vi "Pos Controller.vi"(8 "error in (no error)":errorcluster, 10 "Notifiers":T1, 11 "All Message Queue Cluster":T2) -> (0 "error out":errorcluster)   [LabVIEW 2017]
uses:
  Lib QMH/AllMessageQueue Cluster.ctl
  Lib QMH/Message Cluster.ctl
  Lib Notifier/Notifier.ctl
  Lib QMH/MessageQueues.lvlib
  Lib Log/Logging.lvlib
  Lib Notifier/Notifier.lvlib
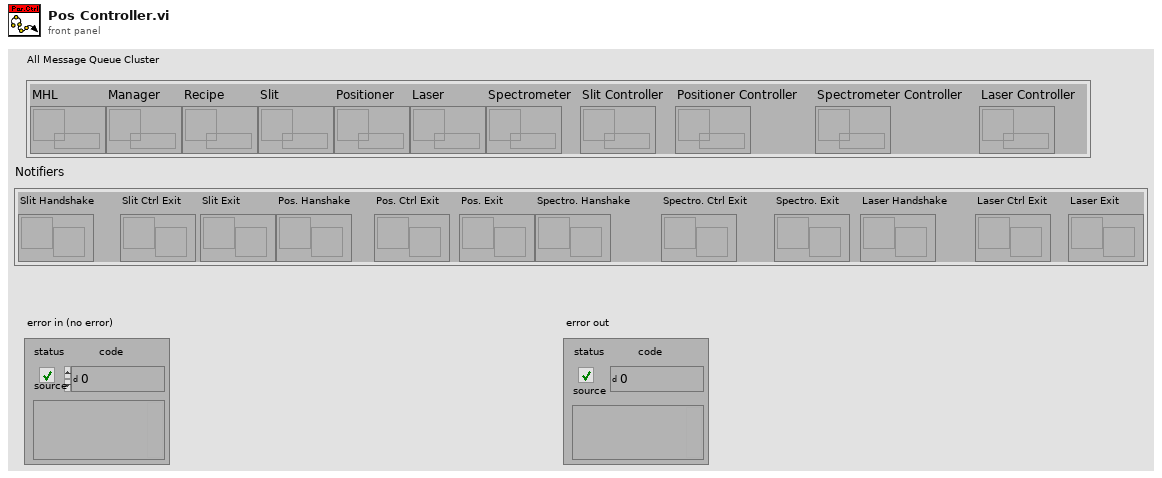
[diagram p1: front panel]
types:
  T1 = typedef "Notifier.lvlib/Notifier.ctl" = cluster{"Slit Handshake":refnum<notifier>, "Slit Ctrl Exit":refnum<notifier>, "Slit Exit":refnum<notifier>, "Pos. Hanshake":refnum<notifier>, "Pos. Ctrl Exit":refnum<notifier>, "Pos. Exit":refnum<notifier>, "Spectro. Hanshake":refnum<notifier>, "Spectro. Ctrl Exit":refnum<notifier>, "Spectro. Exit":refnum<notifier>, "Laser Handshake":refnum<notifier>, "Laser Ctrl Exit":refnum<notifier>, "Laser Exit":refnum<notifier>}
  T2 = typedef "MessageQueues.lvlib/AllMessageQueue Cluster.ctl" = cluster{"MHL":refnum<queue>, "Manager":refnum<queue>, "Recipe":refnum<queue>, "Slit":refnum<queue>, "Positioner":refnum<queue>, "Laser":refnum<queue>, "Spectrometer":refnum<queue>, "Slit Controller":refnum<queue>, "Positioner Controller":refnum<queue>, "Spectrometer Controller":refnum<queue>, "Laser Controller":refnum<queue>}
  T3 = enum16{"open", "replace", "create", "open or create", "replace or create", "replace or create with confirmation"}
  T4 = cluster{"état":bool, "code":i32, "source":string}
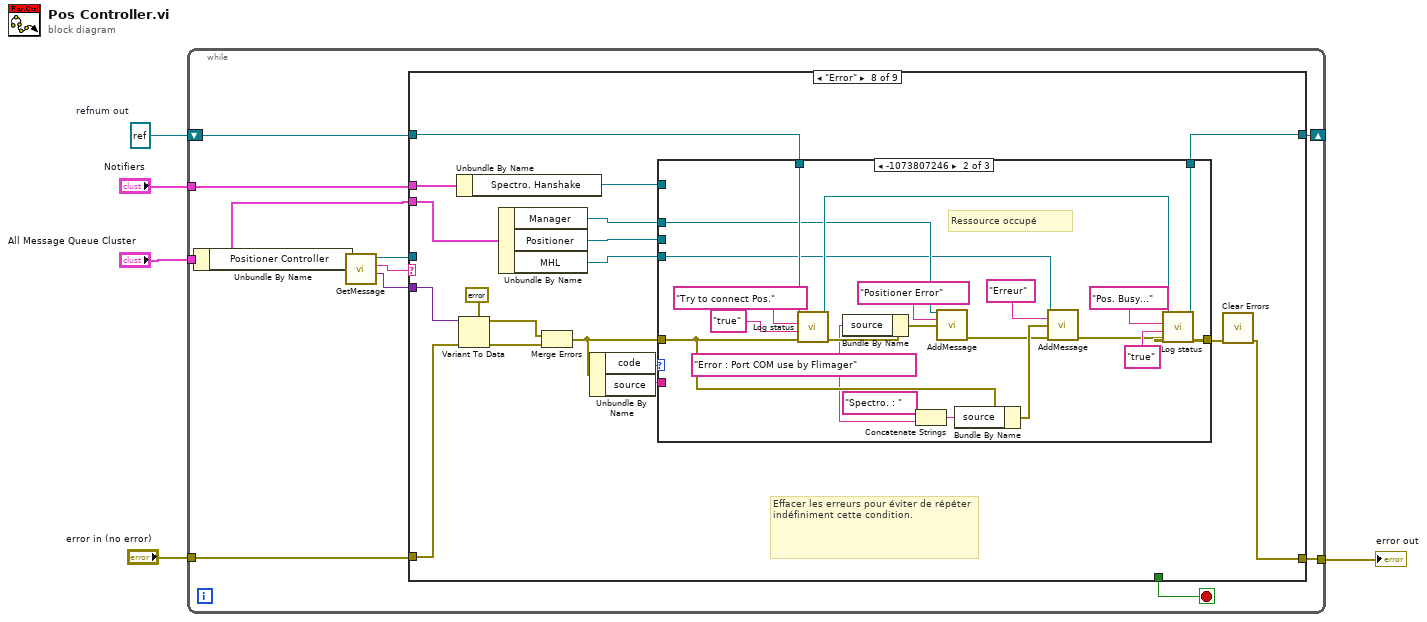
[diagram p0: block diagram]
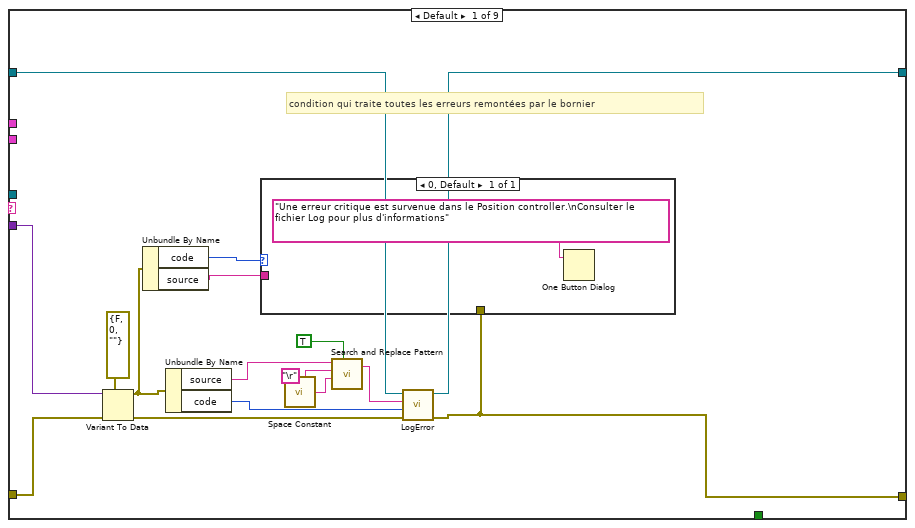
[diagram p2: hidden frame]
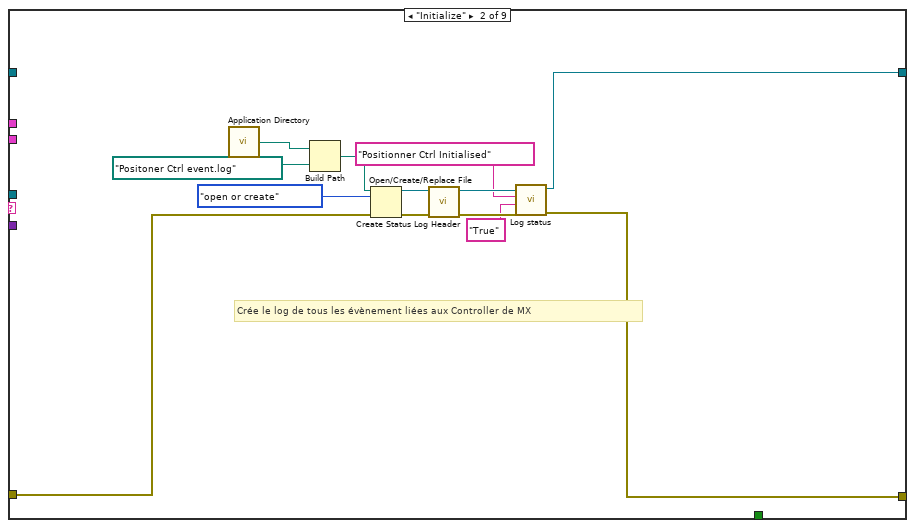
[diagram p3: hidden frame]
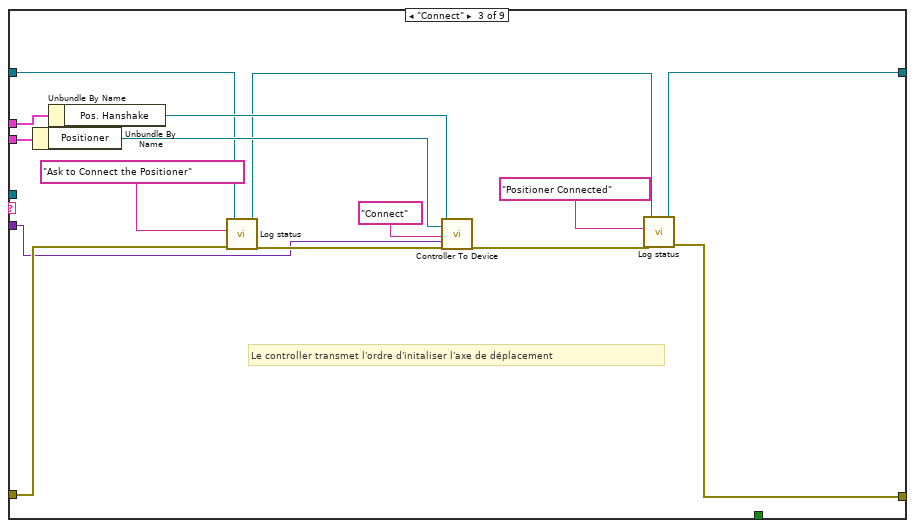
[diagram p4: hidden frame]
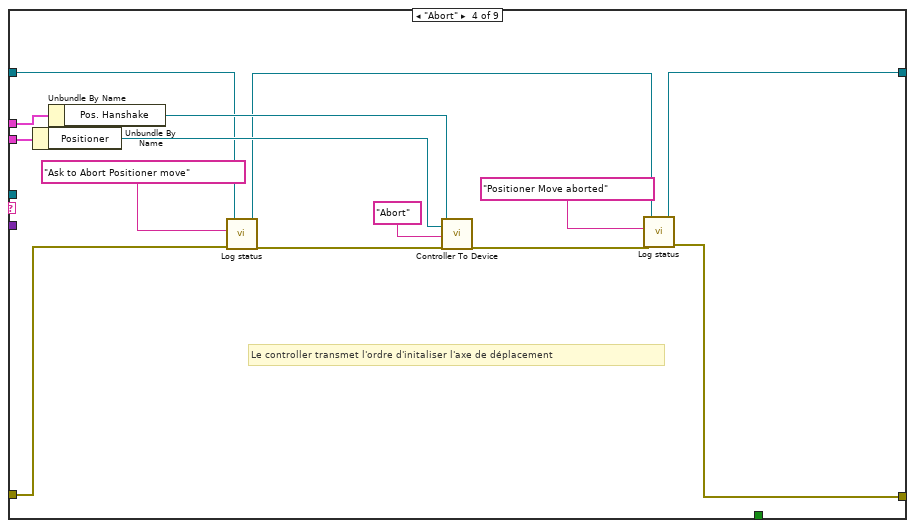
[diagram p5: hidden frame]
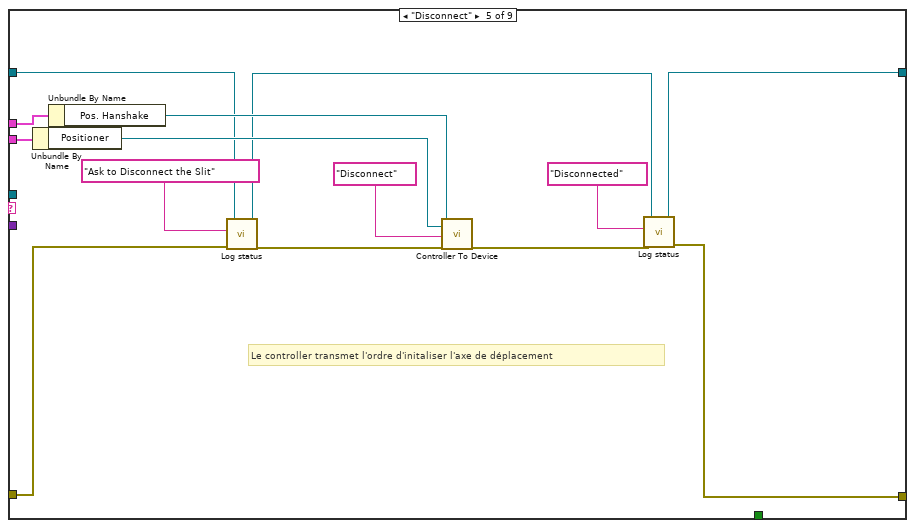
[diagram p6: hidden frame]
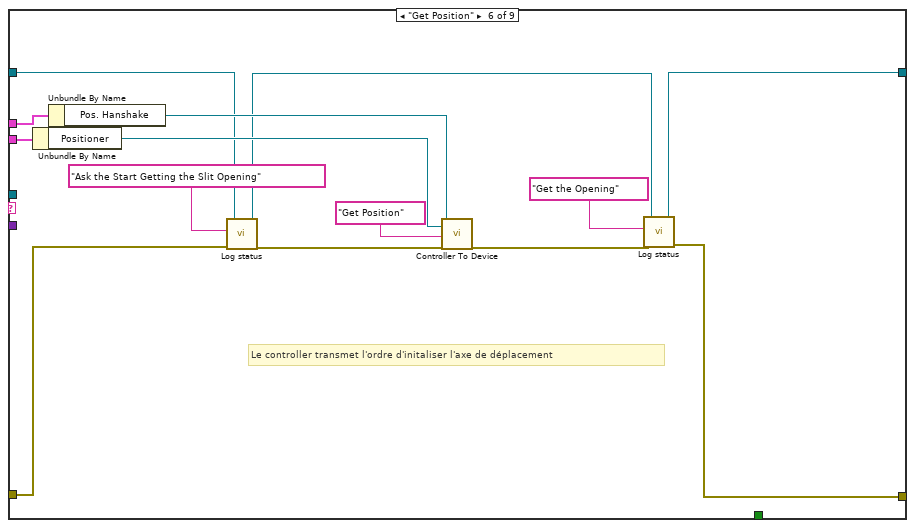
[diagram p7: hidden frame]
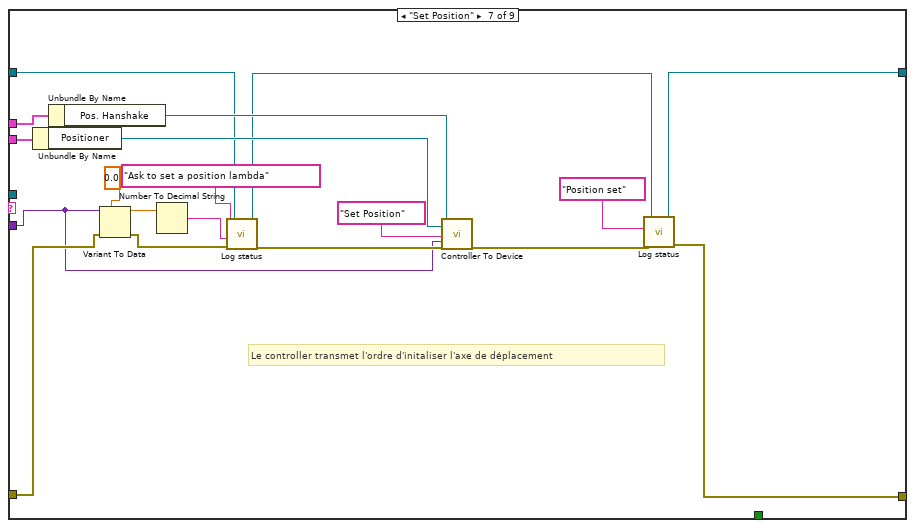
[diagram p8: hidden frame]
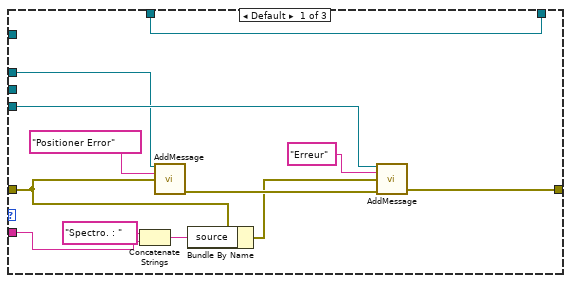
[diagram p9: hidden frame]
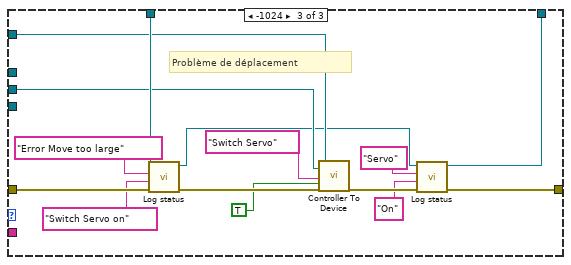
[diagram p10: hidden frame]
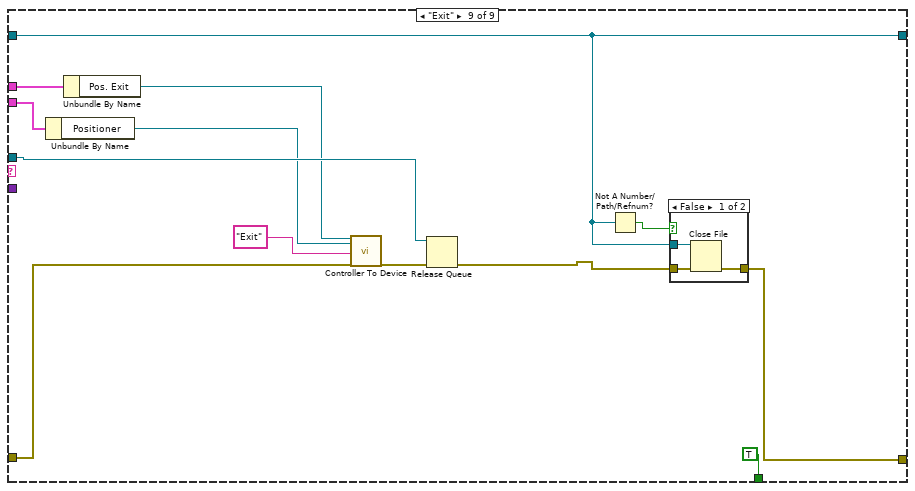
[diagram p11: hidden frame]
diagram:
  w2 = refnum<file> refnum  # refnum out
  n1 = while {
    tunnel: "All Message Queue Cluster" -> [w12]
    tunnel: "Notifiers" -> [w13]
    tunnel: "error in (no error)" -> [w8]
    tunnel: [w6] -> w1
    shift-right: [w14] -> _
    shift-left: w2 -> [w15]
    stop <- w7 stop-if-true
    n2 = Unbundle By Name(w12) -> ("Positioner Controller"=w16:refnum<queue>)
    n3 = call "GetMessage.vi"("Message queue"=w16) -> ("Data"=w9:variant, "Message"=w10:string, "Dup Message Queue"=w11:refnum<queue>)  [unwired: 7 in, 1 out]
    n4 = case shown="\"Error\"" w10 {
      tunnel: w13 -> [_ _ w61 w75 w89 w103 w122 w127 w197]
      tunnel: w12 -> [_ _ w60 w74 w88 w102 w121 w130 w196]
      tunnel: w8 -> [w21 w36 w49 w63 w77 w91 w106 w132 w192]
      tunnel: [_ _ _ _ _ _ _ _ TRUE] -> w7
      tunnel: w11 -> [_ _ _ _ _ _ _ _ w198]
      tunnel: w9 -> [w19 _ w47 _ _ _ w104 w133 _]
      tunnel: [w17 w34 w52 w66 w80 w94 w113 w125 w194] -> w14
      tunnel: w15 -> [w18 _ w56 w70 w84 w98 w117 w128 w194]
      tunnel: [w20 w35 w54 w68 w82 w96 w115 w131 w195] -> w6
      frame Default {
        # "condition qui traite toutes les erreurs remontées par le bornier"
        n5 = Variant To Data(error in=w21, type=errorcluster {"status"=FALSE, "code"=0, "source"=""} ("error in (no error)"), Variant=w19) -> (data=w32:errorcluster, error out=w23:errorcluster)
        n6 = Unbundle By Name(w32) -> ("code"=w30:i32, "source"=w31:string)
        n7 = Unbundle By Name(w32) -> ("source"=w25:string, "code"=w24:i32)
        n8 = call <vilib>:"Space Constant.vi"() -> ("String"=w27:string)
        n9 = call <vilib>:"Search and Replace Pattern.vi"("string"=w25, "regular expression (\"\")"="\r", "replace string (\"\")"=w27, "replace all? (F)"=TRUE) -> ("result string"=w28:string)  [unwired: 1 in, 1 out]
        n10 = call "LogError.vi"("entrée d'erreur"=w23, "Code"=w24, "Source"=w28, "Error log refnum In"=w18) -> ("error out"=w20:errorcluster, "Error log refnum out"=w17:refnum<file>)  [unwired: 6 in]
        n11 = case shown="0, Default" w30 {
          tunnel: w31 -> [_]
          tunnel: w20 -> [_]
          frame 0, Default {
            n12 = One Button Dialog(message="Une erreur critique est survenue dans le Position controller.\nConsulter le fichier Log pour plus d'informations" ("chaîne de format")) -> ()  [unwired: 1 in, 1 out]
          }
        }
      }
      frame "Initialize" {
        # "Crée le log de tous les évènement liées aux Controller de MX"
        n13 = call <vilib>:"Application Directory.vi"() -> ("Application Directory"=w43:path)
        n14 = Build Path(base path=w43, name or relative path=path "Positoner Ctrl event.log") -> (appended path=w45:path)
        n15 = Open/Create/Replace File(file path (use dialog)=w45, error in=w36, operation (0:open)=T3."open or create" ("opération (0 : open)")) -> (refnum out=w41:refnum<file>, error out=w42:errorcluster)  [unwired: 3 in, 1 out]
        n16 = call "Create Status Log Header.vi"("entrée d'erreur"=w42, "Log File Refnum In"=w41) -> ("sortie d'erreur"=w40:errorcluster, "Log File Refnum out"=w39:refnum<file>)  [unwired: 8 in]
        n17 = call "Log status.vi"("entrée d'erreur"=w40, "Event Data String (-)"="True", "Event string"="Positionner Ctrl Initialised", "Log File Refnum In"=w39) -> ("error out"=w35:errorcluster, "Log File Refnum out"=w34:refnum<file>)  [unwired: 6 in]
      }
      frame "Connect" {
        # "Le controller transmet l'ordre d'initaliser l'axe de déplacement"
        n18 = Unbundle By Name(w60) -> ("Positioner"=w58:refnum<queue>)
        n19 = Unbundle By Name(w61) -> ("Pos. Hanshake"=w59:refnum<notifier>)
        n20 = call "Log status.vi"("entrée d'erreur"=w49, "Event string"="Ask to Connect the Positioner", "Log File Refnum In"=w56) -> ("error out"=w57:errorcluster, "Log File Refnum out"=w53:refnum<file>)  [unwired: 7 in]
        n21 = call "Controller To Device.vi"("Notifier"=w59, "Message queue"=w58, "Message"="Connect", "Data"=w47, "entrée d'erreur"=w57) -> ("sortie d'erreur"=w55:errorcluster)  [unwired: 12 in, 2 out]
        n22 = call "Log status.vi"("entrée d'erreur"=w55, "Event string"="Positioner Connected", "Log File Refnum In"=w53) -> ("error out"=w54:errorcluster, "Log File Refnum out"=w52:refnum<file>)  [unwired: 7 in]
      }
      frame "Abort" {
        # "Le controller transmet l'ordre d'initaliser l'axe de déplacement"
        n23 = Unbundle By Name(w74) -> ("Positioner"=w72:refnum<queue>)
        n24 = Unbundle By Name(w75) -> ("Pos. Hanshake"=w73:refnum<notifier>)
        n25 = call "Log status.vi"("entrée d'erreur"=w63, "Event string"="Ask to Abort Positioner move", "Log File Refnum In"=w70) -> ("error out"=w71:errorcluster, "Log File Refnum out"=w67:refnum<file>)  [unwired: 7 in]
        n26 = call "Controller To Device.vi"("Notifier"=w73, "Message queue"=w72, "Message"="Abort", "entrée d'erreur"=w71) -> ("sortie d'erreur"=w69:errorcluster)  [unwired: 13 in, 2 out]
        n27 = call "Log status.vi"("entrée d'erreur"=w69, "Event string"="Positioner Move aborted", "Log File Refnum In"=w67) -> ("error out"=w68:errorcluster, "Log File Refnum out"=w66:refnum<file>)  [unwired: 7 in]
      }
      frame "Disconnect" {
        # "Le controller transmet l'ordre d'initaliser l'axe de déplacement"
        n28 = Unbundle By Name(w88) -> ("Positioner"=w86:refnum<queue>)
        n29 = Unbundle By Name(w89) -> ("Pos. Hanshake"=w87:refnum<notifier>)
        n30 = call "Log status.vi"("entrée d'erreur"=w77, "Event string"="Ask to Disconnect the Slit", "Log File Refnum In"=w84) -> ("error out"=w85:errorcluster, "Log File Refnum out"=w81:refnum<file>)  [unwired: 7 in]
        n31 = call "Controller To Device.vi"("Notifier"=w87, "Message queue"=w86, "Message"="Disconnect", "entrée d'erreur"=w85) -> ("sortie d'erreur"=w83:errorcluster)  [unwired: 13 in, 2 out]
        n32 = call "Log status.vi"("entrée d'erreur"=w83, "Event string"="Disconnected", "Log File Refnum In"=w81) -> ("error out"=w82:errorcluster, "Log File Refnum out"=w80:refnum<file>)  [unwired: 7 in]
      }
      frame "Get Position" {
        # "Le controller transmet l'ordre d'initaliser l'axe de déplacement"
        n33 = Unbundle By Name(w102) -> ("Positioner"=w100:refnum<queue>)
        n34 = Unbundle By Name(w103) -> ("Pos. Hanshake"=w101:refnum<notifier>)
        n35 = call "Log status.vi"("entrée d'erreur"=w91, "Event string"="Ask the Start Getting the Slit Opening", "Log File Refnum In"=w98) -> ("error out"=w99:errorcluster, "Log File Refnum out"=w95:refnum<file>)  [unwired: 7 in]
        n36 = call "Controller To Device.vi"("Notifier"=w101, "Message queue"=w100, "Message"="Get Position", "entrée d'erreur"=w99) -> ("sortie d'erreur"=w97:errorcluster)  [unwired: 13 in, 2 out]
        n37 = call "Log status.vi"("entrée d'erreur"=w97, "Event string"="Get the Opening", "Log File Refnum In"=w95) -> ("error out"=w96:errorcluster, "Log File Refnum out"=w94:refnum<file>)  [unwired: 7 in]
      }
      frame "Set Position" {
        # "Le controller transmet l'ordre d'initaliser l'axe de déplacement"
        n38 = Unbundle By Name(w121) -> ("Positioner"=w119:refnum<queue>)
        n39 = Unbundle By Name(w122) -> ("Pos. Hanshake"=w120:refnum<notifier>)
        n40 = Variant To Data(error in=w106, type=0.0, Variant=w104) -> (data=w108:dbl, error out=w105:errorcluster)
        n41 = Number To Decimal String(number=w108) -> (decimal integer string=w107:string)  [unwired: 1 in]
        n42 = call "Log status.vi"("entrée d'erreur"=w105, "Event Data String (-)"=w107, "Event string"="Ask to set a position lambda", "Log File Refnum In"=w117) -> ("error out"=w118:errorcluster, "Log File Refnum out"=w114:refnum<file>)  [unwired: 6 in]
        n43 = call "Controller To Device.vi"("Notifier"=w120, "Message queue"=w119, "Message"="Set Position", "Data"=w104, "entrée d'erreur"=w118) -> ("sortie d'erreur"=w116:errorcluster)  [unwired: 12 in, 2 out]
        n44 = call "Log status.vi"("entrée d'erreur"=w116, "Event string"="Position set", "Log File Refnum In"=w114) -> ("error out"=w115:errorcluster, "Log File Refnum out"=w113:refnum<file>)  [unwired: 7 in]
      }
      frame "Error" {
        # "Effacer les erreurs pour éviter de répéter indéfiniment cette condition."
        n45 = Unbundle By Name(w127) -> ("Spectro. Hanshake"=w126:refnum<notifier>)
        n46 = Variant To Data(error in=w132, type=T4 {"état"=FALSE, "code"=0, "source"=""} ("sortie d'erreur"), Variant=w133) -> (data=w138:T4, error out=w139:errorcluster)
        n47 = Unbundle By Name(w130) -> ("Manager"=w124:refnum<queue>, "Positioner"=w129:refnum<queue>, "MHL"=w134:refnum<queue>)
        n48 = Merge Errors(w138, w139) -> (w135:errorcluster)
        n49 = Unbundle By Name(w135) -> ("code"=w136:i32, "source"=w123:string)
        n50 = case shown="-1073807246" w136 {
          tunnel: [w150 w166 w179] -> w137
          tunnel: w135 -> [w142 w157 w187]
          tunnel: w134 -> [w152 w156 _]
          tunnel: w129 -> [_ _ w181]
          tunnel: w128 -> [w149 w173 w186]
          tunnel: w126 -> [_ _ w182]
          tunnel: [w149 w168 w174] -> w125
          tunnel: w124 -> [w148 w164 _]
          tunnel: w123 -> [w143 _ _]
          frame Default {
            n51 = Concatenate Strings("Spectro. : " ("string"), w143) -> (w144:string)
            n52 = call "AddMessage.vi"("Message queue"=w148, "Message"="Positioner Error", "Data"=w142) -> ("error out"=w146:errorcluster)  [unwired: 11 in, 1 out]
            n53 = Bundle By Name(cluster=w142, "source"=w144) -> (w141:errorcluster)
            n54 = call "AddMessage.vi"("Message queue"=w152, "Message"="Erreur", "Data"=w141, "entrée d'erreur (pas d'erreur)"=w146) -> ("error out"=w150:errorcluster)  [unwired: 10 in, 1 out]
          }
          frame -1073807246 {
            w154 = "Error : Port COM use by Flimager" ("source")
            # "Ressource occupé"
            n55 = call "Log status.vi"("entrée d'erreur"=w157, "Event Data String (-)"="true", "Event string"="Try to connect Pos.", "Log File Refnum In"=w173) -> ("error out"=w163:errorcluster, "Log File Refnum out"=w165:refnum<file>)  [unwired: 6 in]
            n56 = Bundle By Name(cluster=w163, "source"=w154) -> (w162:errorcluster)
            n57 = Concatenate Strings("Spectro. : " ("string"), w154) -> (w159:string)
            n58 = call "AddMessage.vi"("Message queue"=w164, "Message"="Positioner Error", "Data"=w162) -> ("error out"=w155:errorcluster)  [unwired: 11 in, 1 out]
            n59 = Bundle By Name(cluster=w157, "source"=w159) -> (w158:errorcluster)
            n60 = call "AddMessage.vi"("Message queue"=w156, "Message"="Erreur", "Data"=w158, "entrée d'erreur (pas d'erreur)"=w155) -> ("error out"=w153:errorcluster)  [unwired: 10 in, 1 out]
            n61 = call "Log status.vi"("entrée d'erreur"=w153, "Event Data String (-)"="true", "Event string"="Pos. Busy...", "Log File Refnum In"=w165) -> ("error out"=w166:errorcluster, "Log File Refnum out"=w168:refnum<file>)  [unwired: 6 in]
          }
          frame -1024 {
            # "Problème de déplacement"
            n62 = call "Log status.vi"("entrée d'erreur"=w187, "Event Data String (-)"="Switch Servo on", "Event string"="Error Move too large", "Log File Refnum In"=w186) -> ("error out"=w183:errorcluster, "Log File Refnum out"=w175:refnum<file>)  [unwired: 6 in]
            n63 = call "Controller To Device.vi"("Notifier"=w182, "Message queue"=w181, "Message"="Switch Servo" ("Event Data String (-)"), "Data"=TRUE, "entrée d'erreur"=w183) -> ("sortie d'erreur"=w179:errorcluster)  [unwired: 12 in, 2 out]
            n64 = call "Log status.vi"("Event Data String (-)"="On", "Event string"="Servo", "Log File Refnum In"=w175) -> ("Log File Refnum out"=w174:refnum<file>)  [unwired: 7 in, 1 out]
          }
        }
        n65 = call <vilib>:"Clear Errors.vi"("error in (no error)"=w137) -> ("error out"=w131:errorcluster)  [unwired: 5 in, 1 out]
      }
      frame "Exit" {
        n66 = Unbundle By Name(w196) -> ("Positioner"=w189:refnum<queue>)
        n67 = Unbundle By Name(w197) -> ("Pos. Exit"=w190:refnum<notifier>)
        n68 = call "Controller To Device.vi"("Notifier"=w190, "Message queue"=w189, "Message"="Exit", "entrée d'erreur"=w192) -> ("sortie d'erreur"=w193:errorcluster)  [unwired: 13 in, 2 out]
        n69 = Release Queue(queue=w198, error in (no error)=w193) -> (error out=w188:errorcluster)  [unwired: 1 in, 2 out]
        n70 = Not A Number/Path/Refnum?(number/path/refnum=w194) -> (NaN/Path/Refnum?=w199:bool)
        n71 = case shown="False" w199 {
          tunnel: [w203 w204] -> w195
          tunnel: w188 -> [w202 w204]
          tunnel: w194 -> [w201 _]
          frame False {
            n72 = Close File(refnum=w201, error in=w202) -> (error out=w203:errorcluster)  [unwired: 1 out]
          }
          frame True {
          }
        }
      }
    }
  }
  "error out" <- w1
